vi "Minimum Jerk.vi"(0 "X":dbl, 1 "Xfinal":dbl, 2 "Yfinal":dbl, 3 "Zfinal":dbl, 5 "Vx":dbl, 7 "Y":dbl, 9 "Vy":dbl, 11 "Z":dbl, 12 "Vz":dbl, 13 "current_n":u16, 14 "duration":u16) -> (4 "Pos_dest":dbl[](array[numeric]), 6 "Fx":dbl, 8 "Fy":dbl, 10 "Fz":dbl, 15 "n out":u16)   [LabVIEW 2012]
uses:
  Global_var.vi
panel:
  # "The Minimum Jerk Function \n\n[Updated by Ananda, 2017]"
  # "Minimum jerk formula are based on Hogan/Tamar 1985.\nYou have to basically provide start and destination\nlocations, the movement duration, and current timer."
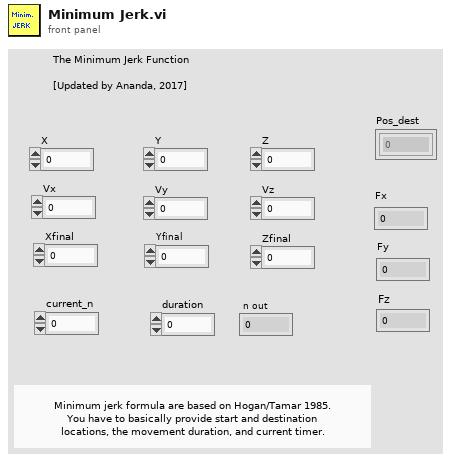
[diagram p1: front panel]
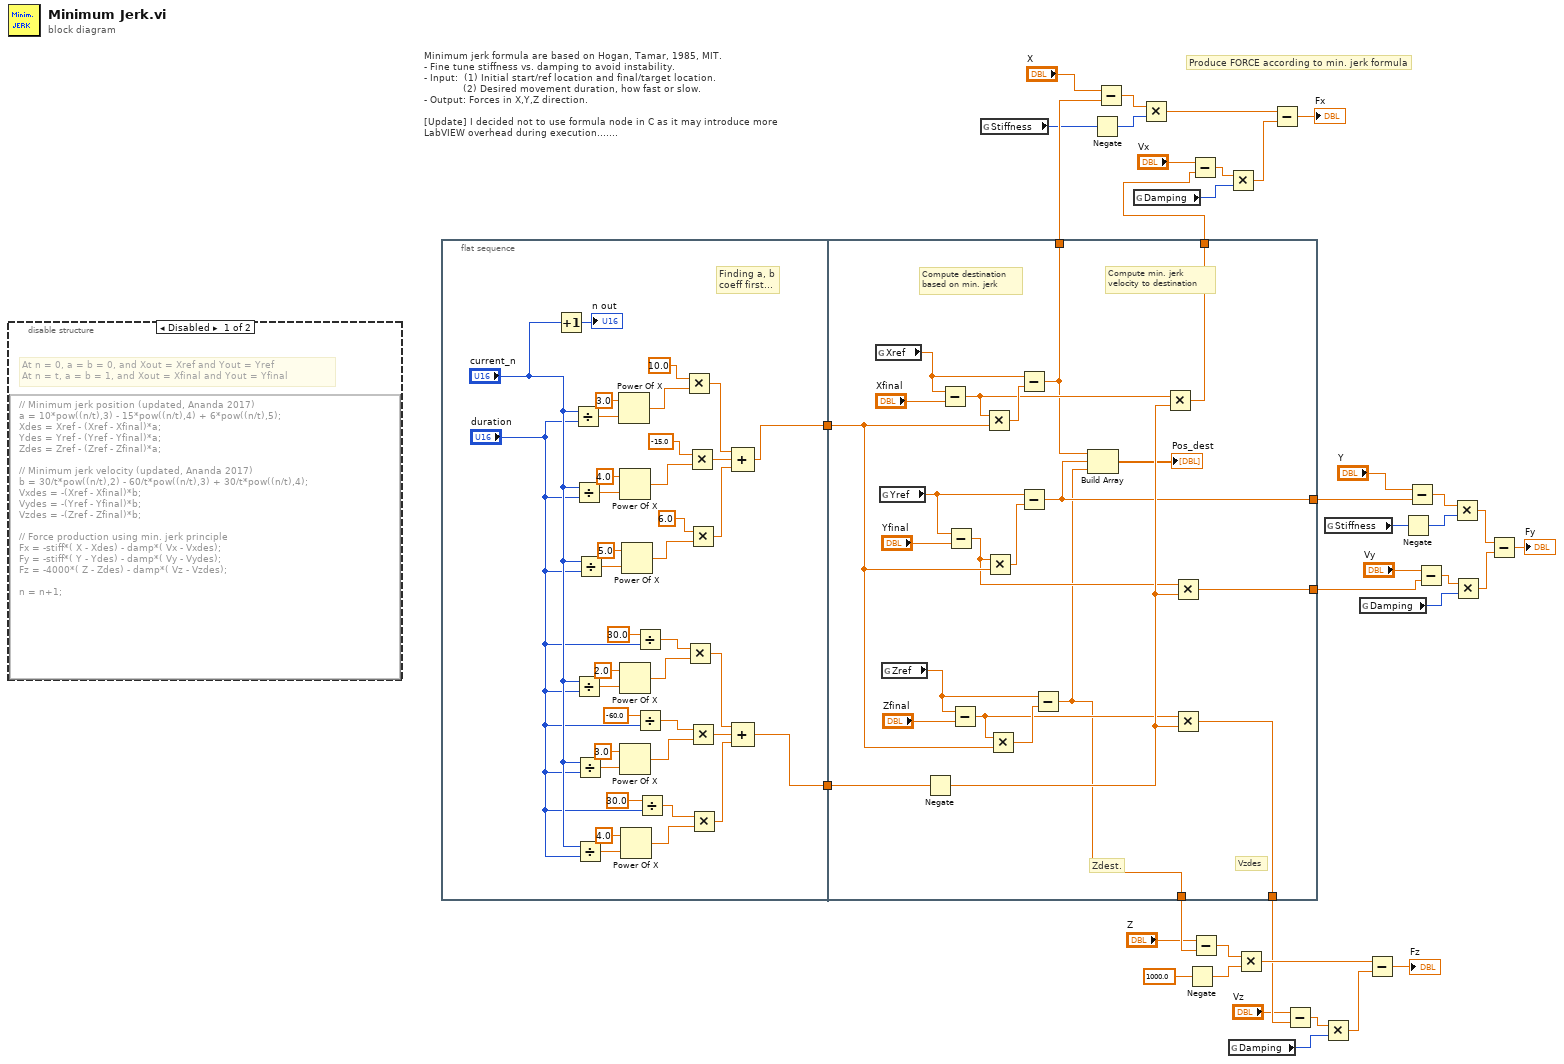
[diagram p0: block diagram]
diagram:
  # "Produce FORCE according to min. jerk formula"
  # "Minimum jerk formula are based on Hogan, Tamar, 1985, MIT.\n- Fine tune stiffness vs. damping to avoid instability.\n- Input:  (1) Initial start/ref location and final/target location.\n             (2) Desired movement duration, how fast or slow.\n- Output: Forces in X,Y,Z direction. \n\n[Update] I decided not to use formula node in C as it may introduce more\nLabVIEW overhead during execution......."
  n1 = disable-structure shown="Disabled" {
    frame Disabled {
      # "At n = 0, a = b = 0, and Xout = Xref and Yout = Yref\nAt n = t, a = b = 1, and Xout = Xfinal and Yout = Yfinal"
      n2 = formula code="// Minimum jerk position (updated, Ananda 2017)\na = 10*pow((n/t),3) - 15*pow((n/t),4) + 6*pow((n/t),5);\nXdes = Xref - (Xref - Xfinal)*a;\nYdes = Yref - (Yref - Yfinal)*a;\nZdes = Zref - (Zref - Zfinal)*a;\n\n// Minimum jerk velocity (updated, Ananda 2017)\nb = 30/t*pow((n/t),2) - 60/t*pow((n/t),3) + 30/t*pow((n/t),4);\nVxdes = -(Xref - Xfinal)*b;\nVydes = -(Yref - Yfinal)*b;\nVzdes = -(Zref - Zfinal)*b;\n\n// Force production using min. jerk principle\nFx = -stiff*( X - Xdes) - damp*( Vx - Vxdes);\nFy = -stiff*( Y - Ydes) - damp*( Vy - Vydes);\nFz = -4000*( Z - Zdes) - damp*( Vz - Vzdes);\n\nn = n+1;"() -> ()
    }
    frame Enabled {
    }
  }
  n3 = flat-sequence {
    tunnel: [w57] -> w38
    tunnel: [w56] -> w37
    tunnel: w38 -> [w95]
    tunnel: w37 -> [w94]
    tunnel: [w80] -> w17
    tunnel: [w83] -> w16
    tunnel: [w78] -> w36
    tunnel: [w81] -> w30
    tunnel: [w82] -> w6
    tunnel: [w79] -> w4
    frame #0 {
      # "Finding a, b\ncoeff first..."
      n4 = Increment(x="current_n") -> (x+1=→"n out":u16)
      n5 = Divide(x="current_n", y="duration") -> (x/y=w55:dbl)
      n6 = Divide(x="current_n", y="duration") -> (x/y=w53:dbl)
      n7 = Divide(x="current_n", y="duration") -> (x/y=w49:dbl)
      n8 = Divide(x="current_n", y="duration") -> (x/y=w47:dbl)
      n9 = Divide(x="current_n", y="duration") -> (x/y=w45:dbl)
      n10 = Divide(x="current_n", y="duration") -> (x/y=w51:dbl)
      n11 = Power Of X(1:w55, 2:3.0 ("x")) -> (0:w75:dbl)
      n12 = Power Of X(1:w53, 2:4.0 ("x")) -> (0:w73:dbl)
      n13 = Power Of X(1:w49, 2:2.0 ("x")) -> (0:w60:dbl)
      n14 = Power Of X(1:w47, 2:3.0 ("x")) -> (0:w62:dbl)
      n15 = Power Of X(1:w45, 2:4.0 ("x")) -> (0:w64:dbl)
      n16 = Power Of X(1:w51, 2:5.0 ("x")) -> (0:w71:dbl)
      n17 = Divide(x=30.0, y="duration") -> (x/y=w43:dbl)
      n18 = Divide(x=-60.0, y="duration") -> (x/y=w41:dbl)
      n19 = Divide(x=30.0, y="duration") -> (x/y=w40:dbl)
      n20 = Multiply(x=10.0, y=w75) -> (x*y=w70:dbl)
      n21 = Multiply(x=w43, y=w60) -> (x*y=w65:dbl)
      n22 = Multiply(x=-15.0, y=w73) -> (x*y=w69:dbl)
      n23 = Multiply(x=6.0, y=w71) -> (x*y=w68:dbl)
      n24 = Multiply(x=w41, y=w62) -> (x*y=w66:dbl)
      n25 = Multiply(x=w40, y=w64) -> (x*y=w67:dbl)
      n26 = Compound Arithmetic op=ADD(w70, w69, w68) -> (w57:dbl)
      n27 = Compound Arithmetic op=ADD(w65, w66, w67) -> (w56:dbl)
    }
    frame #1 {
      # "Vzdes"
      # "Zdest."
      # "Compute min. jerk \nvelocity to destination"
      # "Compute destination\nbased on min. jerk"
      n28 = global read "Global_var.vi" "Xref"() -> (w93:dbl)
      n29 = global read "Global_var.vi" "Yref"() -> (w91:dbl)
      n30 = global read "Global_var.vi" "Zref"() -> (w89:dbl)
      n31 = Negate(x=w94) -> (-x=w86:dbl)
      n32 = Subtract(x=w93, y="Xfinal") -> (x-y=w87:dbl)
      n33 = Subtract(x=w91, y="Yfinal") -> (x-y=w85:dbl)
      n34 = Subtract(x=w89, y="Zfinal") -> (x-y=w84:dbl)
      n35 = Multiply(x=w87, y=w95) -> (x*y=w98:dbl)
      n36 = Multiply(x=w85, y=w95) -> (x*y=w97:dbl)
      n37 = Multiply(x=w84, y=w95) -> (x*y=w96:dbl)
      n38 = Subtract(x=w93, y=w98) -> (x-y=w80:dbl)
      n39 = Subtract(x=w91, y=w97) -> (x-y=w79:dbl)
      n40 = Subtract(x=w89, y=w96) -> (x-y=w78:dbl)
      n41 = Build Array(w80, w79, w78) -> (→"Pos_dest":dbl[])
      n42 = Multiply(x=w87, y=w86) -> (x*y=w83:dbl)
      n43 = Multiply(x=w85, y=w86) -> (x*y=w82:dbl)
      n44 = Multiply(x=w84, y=w86) -> (x*y=w81:dbl)
    }
  }
  n45 = global read "Global_var.vi" "Stiffness"() -> (w2:i16)
  n46 = Negate(x=w2) -> (-x=w19:i16)
  n47 = Subtract(x="X", y=w17) -> (x-y=w20:dbl)
  n48 = global read "Global_var.vi" "Damping"() -> (w25:i16)
  n49 = Multiply(x=w20, y=w19) -> (x*y=w21:dbl)
  n50 = Negate(x=1000.0) -> (-x=w34:dbl)
  n51 = Subtract(x="Vx", y=w16) -> (x-y=w23:dbl)
  n52 = Subtract(x="Z", y=w36) -> (x-y=w33:dbl)
  n53 = Multiply(x=w23, y=w25) -> (x*y=w24:dbl)
  n54 = global read "Global_var.vi" "Damping"() -> (w26:i16)
  n55 = Multiply(x=w33, y=w34) -> (x*y=w32:dbl)
  n56 = Subtract(x=w21, y=w24) -> (x-y=→"Fx":dbl)
  n57 = Subtract(x="Vz", y=w30) -> (x-y=w28:dbl)
  n58 = Multiply(x=w28, y=w26) -> (x*y=w27:dbl)
  n59 = global read "Global_var.vi" "Stiffness"() -> (w1:i16)
  n60 = global read "Global_var.vi" "Damping"() -> (w7:i16)
  n61 = Subtract(x=w32, y=w27) -> (x-y=→"Fz":dbl)
  n62 = Negate(x=w1) -> (-x=w13:i16)
  n63 = Subtract(x="Y", y=w4) -> (x-y=w12:dbl)
  n64 = Subtract(x="Vy", y=w6) -> (x-y=w9:dbl)
  n65 = Multiply(x=w12, y=w13) -> (x*y=w11:dbl)
  n66 = Multiply(x=w9, y=w7) -> (x*y=w8:dbl)
  n67 = Subtract(x=w11, y=w8) -> (x-y=→"Fy":dbl)
